vi "addDataSGL.vi"(8 "error in (no error)":errorcluster, 9 "OverrideSwapBytes":bool, 10 "Data":sgl, 11 "U8ArrayBuilderAutoIndexing in":refnum<class "U8ArrayBuilderAutoIndexing.lvclass">) -> (0 "error out":errorcluster, 3 "U8ArrayBuilderAutoIndexing out":refnum<class "U8ArrayBuilderAutoIndexing.lvclass">)   [LabVIEW 2016, in "RTUtilities.lvlib" / "U8ArrayBuilderAutoIndexing.lvclass"]
uses:
  U8ArrayBuilderAutoIndexing.lvclass
  U8ArrayBuilderAutoIndexing.lvclass/U8ArrayBuilderAutoIndexing.ctl
  U8ArrayBuilderManualIndexing/U8ArrayBuilderManualIndexing.lvclass
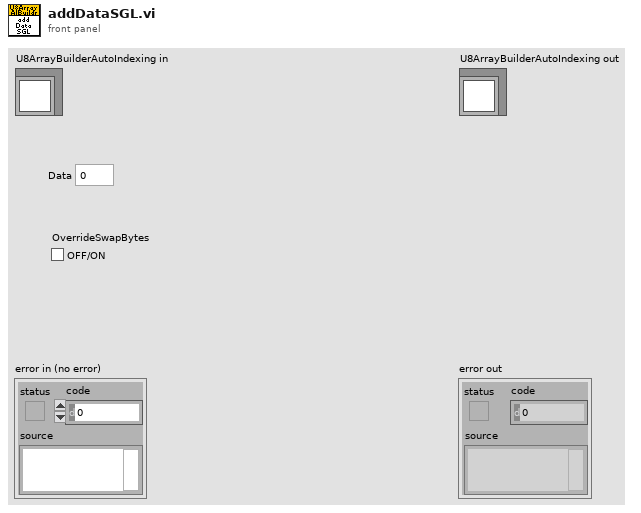
[diagram p1: front panel]
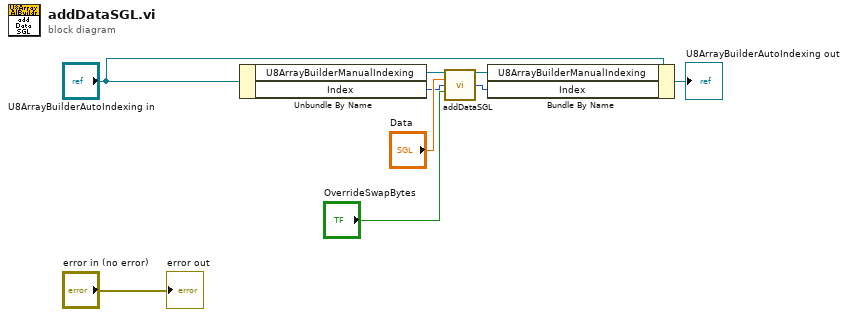
[diagram p0: block diagram]
diagram:
  n1 = Unbundle By Name("U8ArrayBuilderAutoIndexing in") -> ("U8ArrayBuilderManualIndexing"=w7:refnum<class "U8ArrayBuilderManualIndexing.lvclass">, "Index"=w5:i32)
  n2 = call "addDataSGL.vi"("U8ArrayBuilderManualIndexing in"=w7, "Data"="Data", "Index"=w5, "OverrideSwapBytes"="OverrideSwapBytes") -> ("U8ArrayBuilderManualIndexing out"=w2:refnum<class "U8ArrayBuilderManualIndexing.lvclass">, "Index out"=w3:i32)  [unwired: 9 in, 1 out]
  n3 = Bundle By Name(cluster="U8ArrayBuilderAutoIndexing in", "U8ArrayBuilderManualIndexing"=w2, "Index"=w3) -> (→"U8ArrayBuilderAutoIndexing out":refnum<class "U8ArrayBuilderAutoIndexing.lvclass">)
  "error out" <- "error in (no error)"
